vi "多步计算.vi"(0 "输入棋盘状态":i32[][](array[numeric])) -> (4 "输出棋盘状态":i32[][](array[numeric]), 6 "最佳的行":sgl, 8 "最佳的列":i16)   [LabVIEW 2018]
panel:
  in  "搜索深度":i8=2
  out "列":i16
  out "行":sgl
  out "当前列":i16
  out "当前行":sgl
  out "权值最大的三个位置":dbl[][](array[numeric])
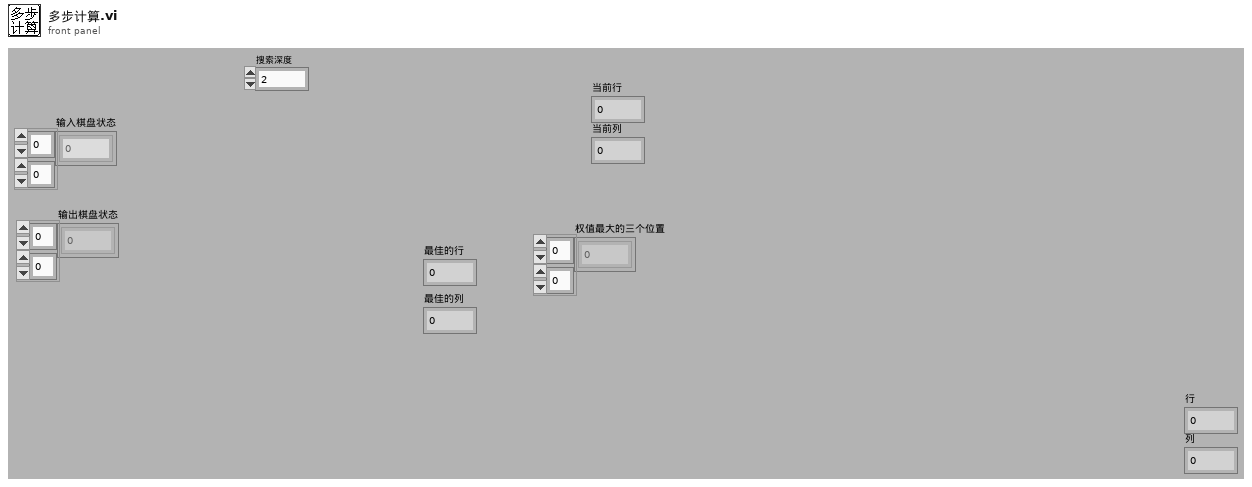
[diagram p1: front panel]
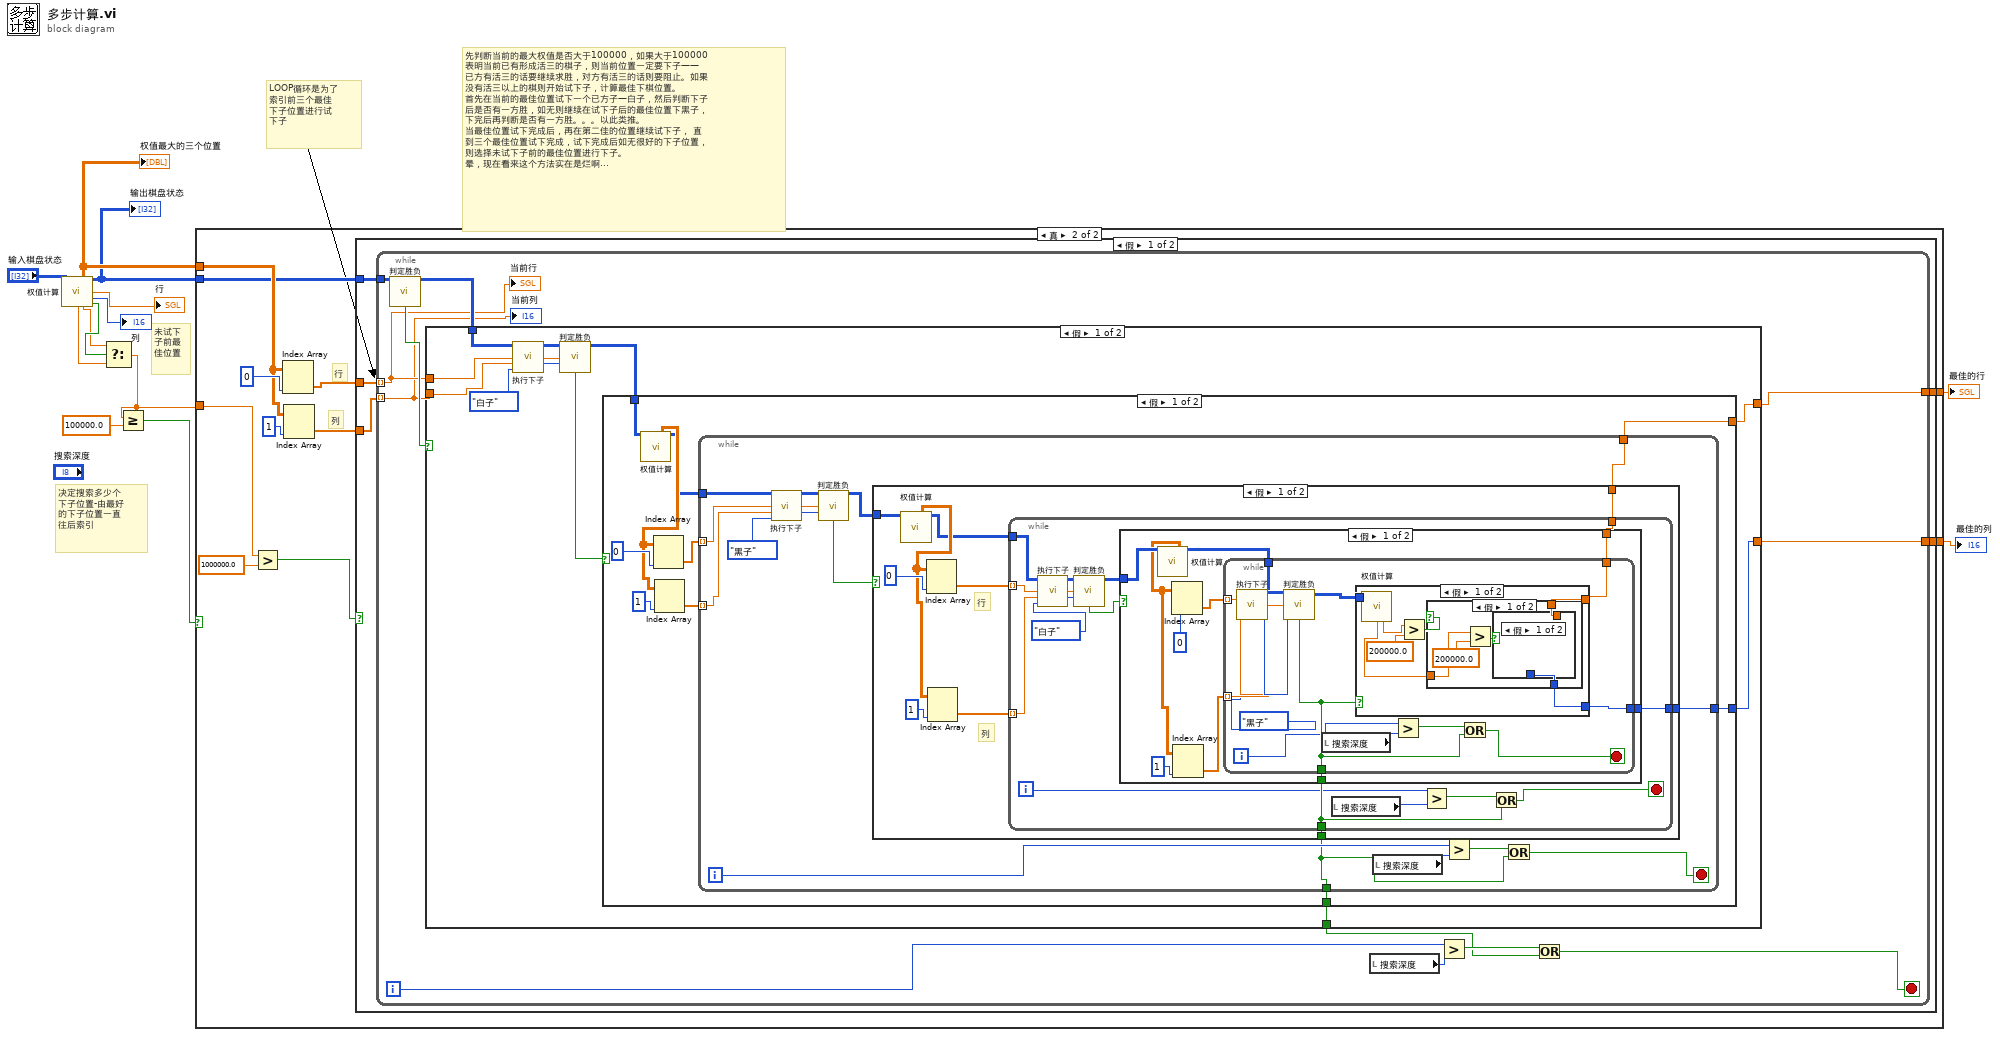
[diagram p0: block diagram]
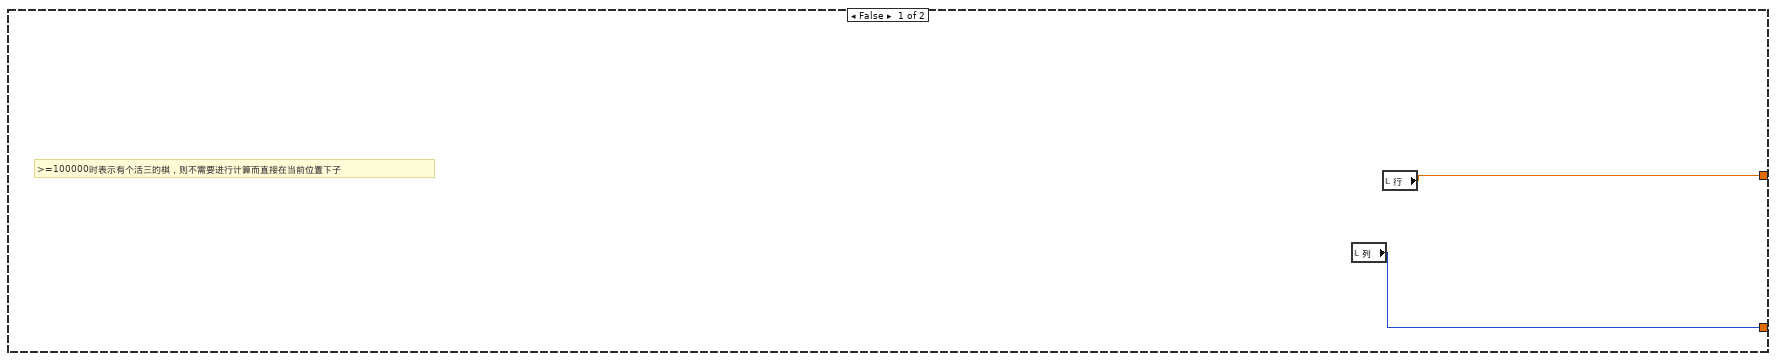
[diagram p2: hidden frame]
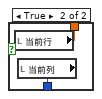
[diagram p3: hidden frame]
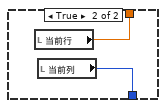
[diagram p4: hidden frame]
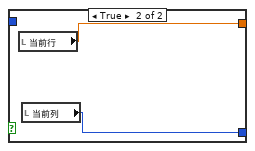
[diagram p5: hidden frame]
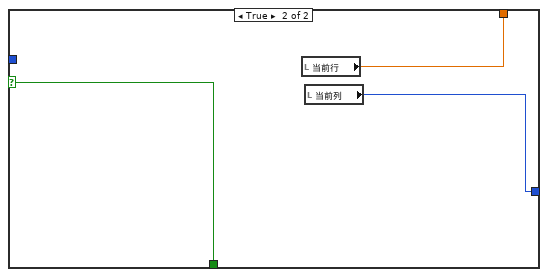
[diagram p6: hidden frame]
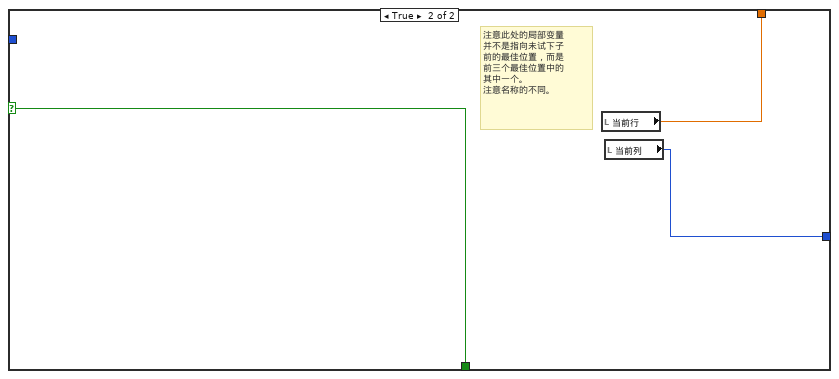
[diagram p7: hidden frame]
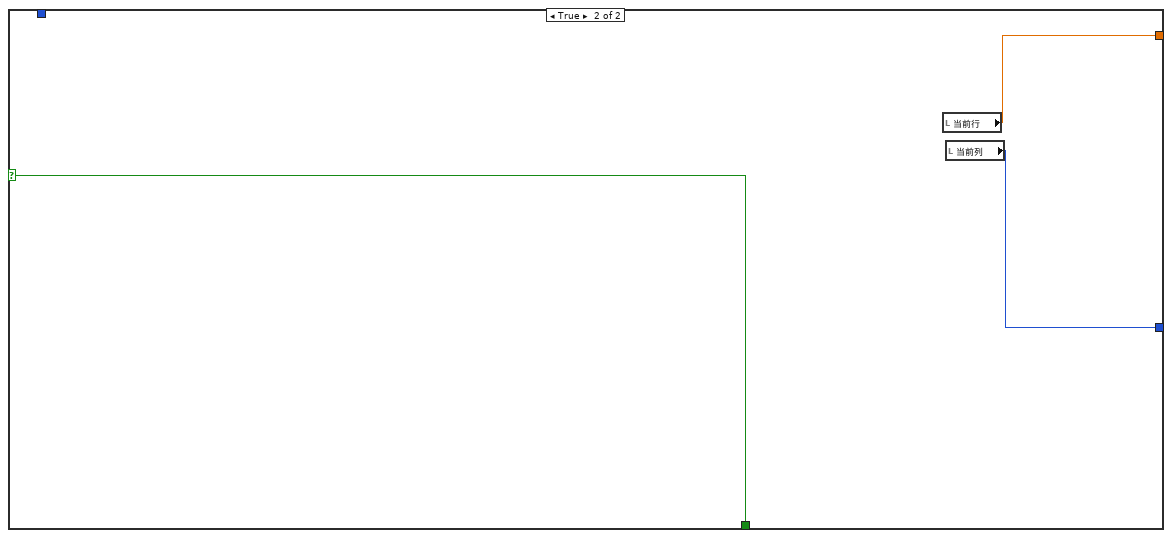
[diagram p8: hidden frame]
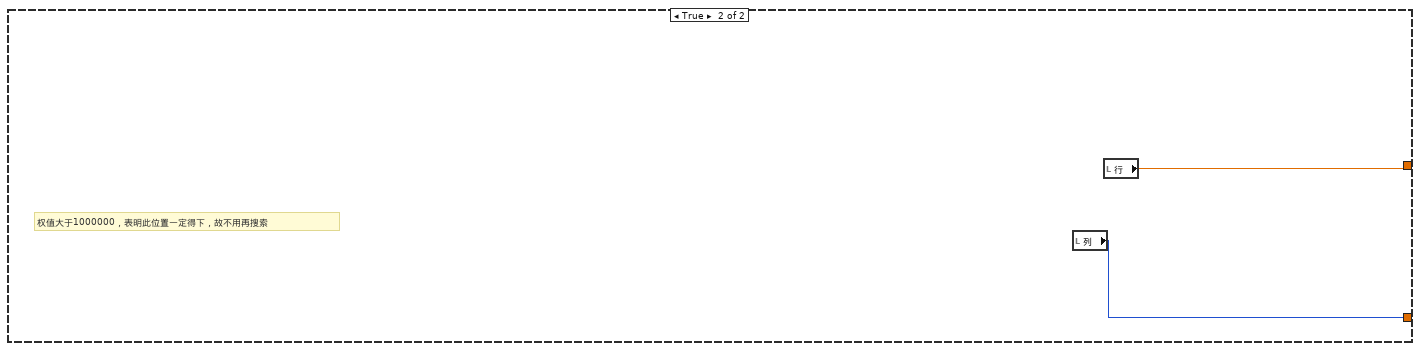
[diagram p10: hidden frame]
diagram:
  # "决定搜索多少个\n下子位置-由最好\n的下子位置一直\n往后索引"
  # "LOOP循环是为了\n索引前三个最佳\n下子位置进行试\n下子"
  # "未试下\n子前最\n佳位置"
  # "先判断当前的最大权值是否大于100000，如果大于100000\n表明当前已有形成活三的棋子，则当前位置一定要下子——\n已方有活三的话要继续求胜，对方有活三的话则要阻止。如果\n没有活三以上的棋则开始试下子，计算最佳下棋位置。\n首先在当前的最佳位置试下一个已方子—白子，然后判断下子\n后是否有一方胜，如无则继续在试下子后的最佳位置下黑子，\n下完后再判断是否有一方胜。。。以此类推。\n当最佳位置试下完成后，再在第二佳的位置继续试下子， 直\n到三个最佳位置试下完成，试下完成后如无很好的下子位置，\n则选择未试下子前的最佳位置进行下子。\n晕，现在看来这个方法实在是烂啊..."
  n1 = call "权值计算.vi"("当前棋盘状态"="输入棋盘状态") -> ("权值最大的三个位置"=w12:dbl[][], "当前棋盘状态"=w9:i32[][], "行"=→"行":sgl, "列"=→"列":i16, "黑子最大权值"=w4:sgl, "白子最大权值"=w5:sgl, "白子权值大于黑子？"=w6:bool)  [unwired: 8 in]
  "输出棋盘状态" <- w9
  "权值最大的三个位置" <- w12
  n2 = Select(t=w5, s=w6, f=w4) -> (s? t:f=w1:sgl)
  n3 = Greater Or Equal?(x=w1, y=sgl 100000.0) -> (x >= y?=w2:bool)
  n4 = case shown="真" w2 {
    tunnel: w12 -> [_ w25]
    tunnel: [w15 w22] -> w11
    tunnel: [w14 w21] -> w10
    tunnel: w9 -> [_ w19]
    tunnel: w1 -> [_ w18]
    frame False {
      # ">=100000时表示有个活三的棋，则不需要进行计算而直接在当前位置下子"
      n5 = local read "列"() -> (w14:i16)
      n6 = local read "行"() -> (w15:sgl)
    }
    frame True {
      # "列"
      # "行"
      n7 = Greater?(x=w18, y=sgl 1000000.0) -> (0:w16:bool)
      n8 = Index Array(array=w25, index (col)=0 ("index (row)")) -> (element=w20:dbl[])  [unwired: 1 in]
      n9 = Index Array(array=w25, index (col)=1 ("index (row)")) -> (element=w23:dbl[])  [unwired: 1 in]
      n10 = case shown="假" w16 {
        tunnel: w23 -> [w31 _]
        tunnel: [w30 w166] -> w22
        tunnel: [w29 w165] -> w21
        tunnel: w20 -> [w28 _]
        tunnel: w19 -> [w27 _]
        frame False {
          n11 = while {
            tunnel: w28 -> [w38] mode=indexing
            tunnel: w31 -> [w37] mode=indexing
            tunnel: [w43] -> w30
            tunnel: [w42] -> w29
            tunnel: w27 -> [w41]
            i -> [w34]
            stop <- w32 stop-if-true
            n12 = call "判定胜负.vi"("当前棋盘状态"=w41) -> ("当前棋盘状态"=w39:i32[][], "此局结束?"=w40:bool)  [unwired: 9 in, 4 out]
            n13 = case shown="假" w40 {
              selector: w40 -> [_ w162]
              tunnel: w38 -> [w51 w164]
              tunnel: w37 -> [w50 w163]
              tunnel: [w46 w164] -> w43
              tunnel: [w45 w163] -> w42
              tunnel: w39 -> [w49 _]
              tunnel: [w44 w162] -> w33
              frame False {
                n14 = call "执行下子.vi"("当前棋盘状态"=w49, "行"=w51, "列"=w50, "白子/黑子?"=enum16{"白子", "无子", "黑子"}."白子") -> ("当前棋盘状态"=w53:i32[][], "行"=w54:sgl, "列"=w55:i16)  [unwired: 8 in, 1 out]
                n15 = call "判定胜负.vi"("当前棋盘状态"=w53, "行"=w54, "列"=w55) -> ("当前棋盘状态"=w47:i32[][], "此局结束?"=w48:bool)  [unwired: 7 in, 4 out]
                n16 = case shown="假" w48 {
                  selector: w48 -> [_ w159]
                  tunnel: w47 -> [w65 _]
                  tunnel: [w58 w161] -> w46
                  tunnel: [w57 w160] -> w45
                  tunnel: [w56 w159] -> w44
                  frame False {
                    n17 = call "权值计算.vi"("当前棋盘状态"=w65) -> ("权值最大的三个位置"=w62:dbl[][], "当前棋盘状态"=w59:i32[][])  [unwired: 8 in, 5 out]
                    n18 = Index Array(array=w62, index (col)=0 ("index (row)")) -> (element=w61:dbl[])  [unwired: 1 in]
                    n19 = Index Array(array=w62, index (col)=1 ("index (row)")) -> (element=w60:dbl[])  [unwired: 1 in]
                    n20 = while {
                      tunnel: w61 -> [w76] mode=indexing
                      tunnel: w60 -> [w75] mode=indexing
                      tunnel: w59 -> [w78]
                      tunnel: [w72] -> w58
                      tunnel: [w71] -> w57
                      tunnel: [w66] -> w56
                      i -> [w67]
                      stop <- w68 stop-if-true
                      n21 = call "执行下子.vi"("当前棋盘状态"=w78, "行"=w76, "列"=w75, "白子/黑子?"=enum16{"白子", "无子", "黑子"}."黑子") -> ("当前棋盘状态"=w77:i32[][], "行"=w81:sgl, "列"=w80:i16)  [unwired: 8 in, 1 out]
                      n22 = call "判定胜负.vi"("当前棋盘状态"=w77, "行"=w81, "列"=w80) -> ("当前棋盘状态"=w73:i32[][], "此局结束?"=w74:bool)  [unwired: 7 in, 4 out]
                      n23 = case shown="假" w74 {
                        selector: w74 -> [_ w156]
                        tunnel: w73 -> [w91 _]
                        tunnel: [w84 w158] -> w72
                        tunnel: [w83 w157] -> w71
                        tunnel: [w82 w156] -> w66
                        frame False {
                          # "列"
                          # "行"
                          n24 = call "权值计算.vi"("当前棋盘状态"=w91) -> ("权值最大的三个位置"=w88:dbl[][], "当前棋盘状态"=w85:i32[][])  [unwired: 8 in, 5 out]
                          n25 = Index Array(array=w88, index (col)=0 ("index (row)")) -> (element=w87:dbl[])  [unwired: 1 in]
                          n26 = Index Array(array=w88, index (col)=1 ("index (row)")) -> (element=w86:dbl[])  [unwired: 1 in]
                          n27 = while {
                            tunnel: w87 -> [w102] mode=indexing
                            tunnel: w86 -> [w103] mode=indexing
                            tunnel: w85 -> [w101]
                            tunnel: [w98] -> w84
                            tunnel: [w97] -> w83
                            tunnel: [w93] -> w82
                            i -> [w92]
                            stop <- w94 stop-if-true
                            n28 = call "执行下子.vi"("当前棋盘状态"=w101, "行"=w102, "列"=w103, "白子/黑子?"=enum16{"白子", "无子", "黑子"}."白子") -> ("当前棋盘状态"=w107:i32[][], "行"=w104:sgl, "列"=w105:i16)  [unwired: 8 in, 1 out]
                            n29 = call "判定胜负.vi"("当前棋盘状态"=w107, "行"=w104, "列"=w105) -> ("当前棋盘状态"=w99:i32[][], "此局结束?"=w100:bool)  [unwired: 7 in, 4 out]
                            n30 = case shown="假" w100 {
                              selector: w100 -> [_ w153]
                              tunnel: w99 -> [w117 _]
                              tunnel: [w110 w155] -> w98
                              tunnel: [w109 w154] -> w97
                              tunnel: [w108 w153] -> w93
                              frame False {
                                n31 = call "权值计算.vi"("当前棋盘状态"=w117) -> ("权值最大的三个位置"=w114:dbl[][], "当前棋盘状态"=w111:i32[][])  [unwired: 8 in, 5 out]
                                n32 = Index Array(array=w114, index (col)=0 ("index (row)")) -> (element=w113:dbl[])  [unwired: 1 in]
                                n33 = Index Array(array=w114, index (col)=1 ("index (row)")) -> (element=w112:dbl[])  [unwired: 1 in]
                                n34 = while {
                                tunnel: w113 -> [w129] mode=indexing
                                tunnel: w112 -> [w128] mode=indexing
                                tunnel: w111 -> [w126]
                                tunnel: [w125] -> w110
                                tunnel: [w124] -> w109
                                tunnel: [w122] -> w108
                                i -> [w121]
                                stop <- w119 stop-if-true
                                n35 = call "执行下子.vi"("当前棋盘状态"=w126, "行"=w129, "列"=w128, "白子/黑子?"=enum16{"白子", "无子", "黑子"}."黑子") -> ("当前棋盘状态"=w130:i32[][], "行"=w132:sgl, "列"=w131:i16)  [unwired: 8 in, 1 out]
                                n36 = call "判定胜负.vi"("当前棋盘状态"=w130, "行"=w132, "列"=w131) -> ("当前棋盘状态"=w123:i32[][], "此局结束?"=w122:bool)  [unwired: 7 in, 4 out]
                                n37 = local read "搜索深度"() -> (w118:i8)
                                n38 = case shown="假" w122 {
                                tunnel: [w135 w152] -> w125
                                tunnel: [w134 w151] -> w124
                                tunnel: w123 -> [w139 _]
                                frame False {
                                n39 = call "权值计算.vi"("当前棋盘状态"=w139) -> ("黑子最大权值"=w133:sgl, "白子最大权值"=w138:sgl)  [unwired: 8 in, 5 out]
                                n40 = Greater?(x=w138, y=sgl 200000.0) -> (0:w136:bool)
                                n41 = case shown="假" w136 {
                                tunnel: [w141 w150] -> w135
                                tunnel: [w140 w149] -> w134
                                tunnel: w133 -> [w143 _]
                                frame False {
                                n42 = Greater?(x=w143, y=sgl 200000.0) -> (0:w142:bool)
                                n43 = case shown="假" w142 {
                                tunnel: [w145 w148] -> w141
                                tunnel: [w146 w147] -> w140
                                frame False {
                                n44 = local read "列"() -> (w146:i16)
                                n45 = local read "行"() -> (w145:sgl)
                                }
                                frame True {
                                n46 = local read "当前行"() -> (w148:sgl)
                                n47 = local read "当前列"() -> (w147:i16)
                                }
                                }
                                }
                                frame True {
                                n48 = local read "当前行"() -> (w150:sgl)
                                n49 = local read "当前列"() -> (w149:i16)
                                }
                                }
                                }
                                frame True {
                                n50 = local read "当前行"() -> (w152:sgl)
                                n51 = local read "当前列"() -> (w151:i16)
                                }
                                }
                                n52 = Greater?(x=w121, y=w118) -> (0:w120:bool)
                                n53 = Or(x=w120, y=w122) -> (x .or. y?=w119:bool)
                                }
                              }
                              frame True {
                                n54 = local read "当前行"() -> (w155:sgl)
                                n55 = local read "当前列"() -> (w154:i16)
                              }
                            }
                            n56 = local read "搜索深度"() -> (w96:i8)
                            n57 = Greater?(x=w92, y=w96) -> (0:w95:bool)
                            n58 = Or(x=w95, y=w93) -> (x .or. y?=w94:bool)
                          }
                        }
                        frame True {
                          # "注意此处的局部变量\n并不是指向未试下子\n前的最佳位置，而是\n前三个最佳位置中的\n其中一个。\n注意名称的不同。"
                          n59 = local read "当前行"() -> (w158:sgl)
                          n60 = local read "当前列"() -> (w157:i16)
                        }
                      }
                      n61 = local read "搜索深度"() -> (w69:i8)
                      n62 = Greater?(x=w67, y=w69) -> (0:w70:bool)
                      n63 = Or(x=w70, y=w66) -> (x .or. y?=w68:bool)
                    }
                  }
                  frame True {
                    n64 = local read "当前行"() -> (w161:sgl)
                    n65 = local read "当前列"() -> (w160:i16)
                  }
                }
              }
              frame True {
                # "有一方胜，则表明当前位置的下子的话就有可能让一方胜，\n不论是哪一方胜都要在此位置下子——\n如果是已方胜，则表明在此位置下自己最有可能\n胜，则要在此位置下；\n如果是对方胜，则表明对方在此位置下时自己\n最有可能输，则也要在此位置下。"
              }
            }
            n66 = local read "搜索深度"() -> (w36:i8)
            n67 = Greater?(x=w34, y=w36) -> (0:w35:bool)
            n68 = Or(x=w35, y=w33) -> (x .or. y?=w32:bool)
            "当前行" <- w38
            "当前列" <- w37
          }
        }
        frame True {
          # "权值大于1000000，表明此位置一定得下，故不用再搜索"
          n69 = local read "列"() -> (w165:i16)
          n70 = local read "行"() -> (w166:sgl)
        }
      }
    }
  }
  "最佳的行" <- w11
  "最佳的列" <- w10
